vi "VAttrbutesToData.vi"(6 "to lowercase?(F)":bool, 7 "Prototype":variant, 8 "error in (no error)":errorcluster, 11 "VAttributes":variant) -> (0 "error out":errorcluster, 3 "data":variant)   [LabVIEW 2019, in "lv-apt-json-file.lvlib"]
uses:
  lv-apt-json-file.lvlib
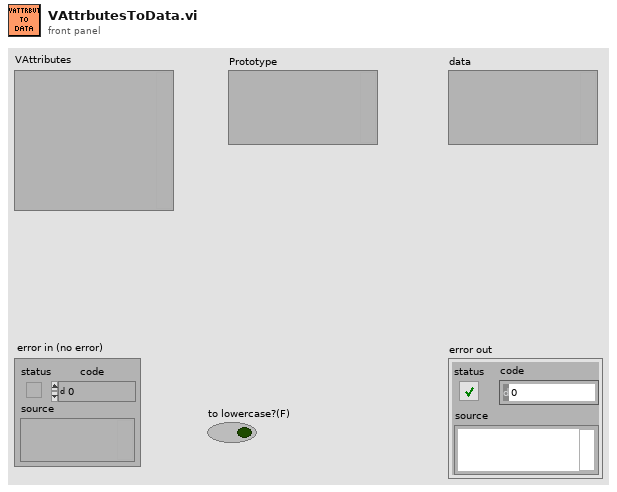
[diagram p1: front panel]
types:
  T1 = typedef "Type Descriptor Enumeration__ogtk.ctl" = enum8{"<Null>", "I8", "I16", "I32", "I64", "U8", "U16", "U32", "U64", "SGL", "DBL", "EXT", "CSG", "CDB", "CXT", "0x0F", "0x10", "0x11", "0x12", "0x13", "0x14", "Enum U8", "Enum U16", "Enum U32", "Enum U64", "SGL PQ", "DBL PQ", "EXT PQ", "CSG PQ", "CDB PQ", "CXT PQ", "0x1F", "0x20", "Boolean", "0x22", "0x23", "0x24", "0x25", "0x26", "0x27", "0x28", "0x29", "0x2A", "0x2B", "0x2C", "0x2D", "0x2E", "0x2F", "String", "0x31", "Path", "Pict", "0x34", "0x35", "0x36", "DAQ", "0x38", "0x39", "0x3A", "0x3B", "0x3C", "0x3D", "0x3E", "0x3F", "Array", "0x41", "0x42", "0x43", "0x44", "0x45", "0x46", "0x47", "0x48", "0x49", "0x4A", "0x4B", "0x4C", "0x4D", "0x4E", "0x4F", "Cluster", "0x51", "0x52", "Variant", "Waveform", "0x55", "0x56", "0x57", "0x58", "0x59", "0x5A", "0x5B", "0x5C", "0x5D", "0x5E", "Fixed Point", "0x60", "0x61", "0x62", "0x63", "0x64", "0x65", "0x66", "0x67", "0x68", "0x69", "0x6A", "0x6B", "0x6C", "0x6D", "0x6E", "0x6F", "Refnum", "0x71", "0x72", "Set Collection", "Map Collection"}
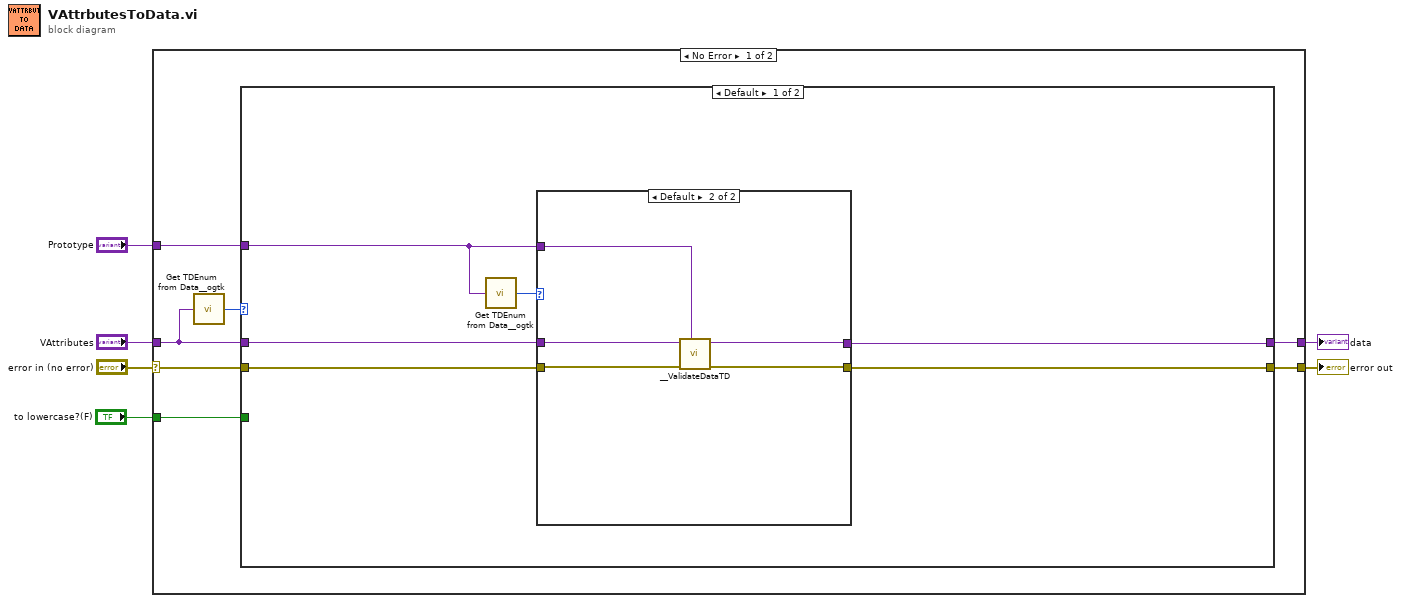
[diagram p0: block diagram]
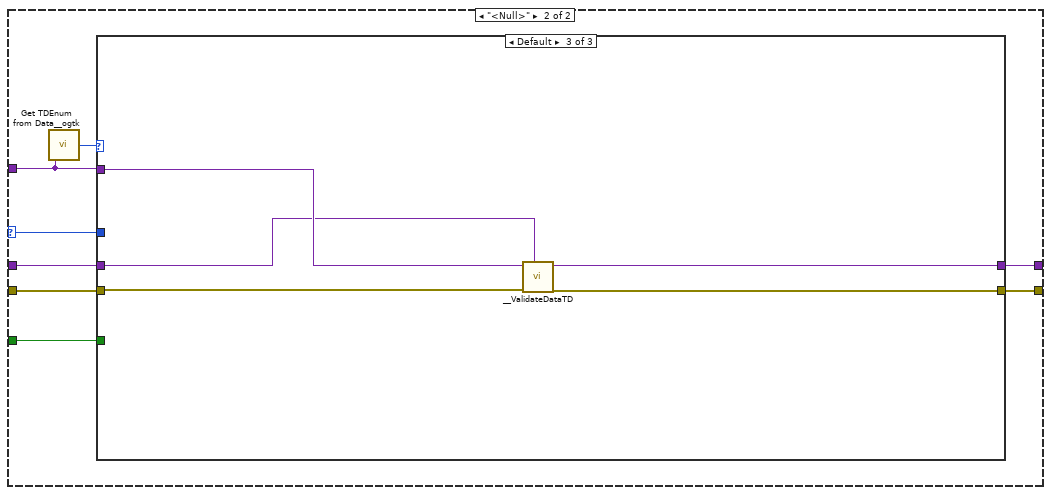
[diagram p3: hidden frame]
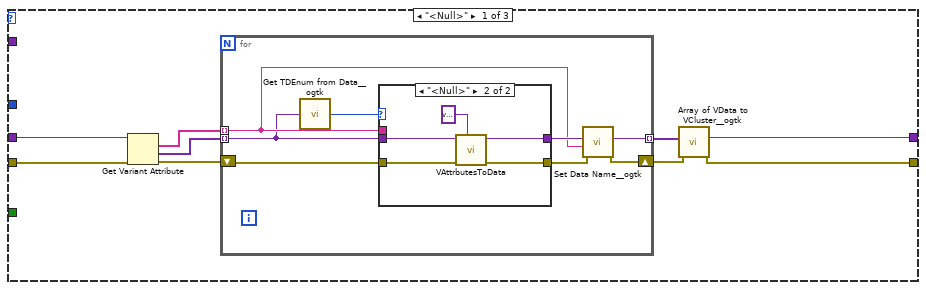
[diagram p4: hidden frame]
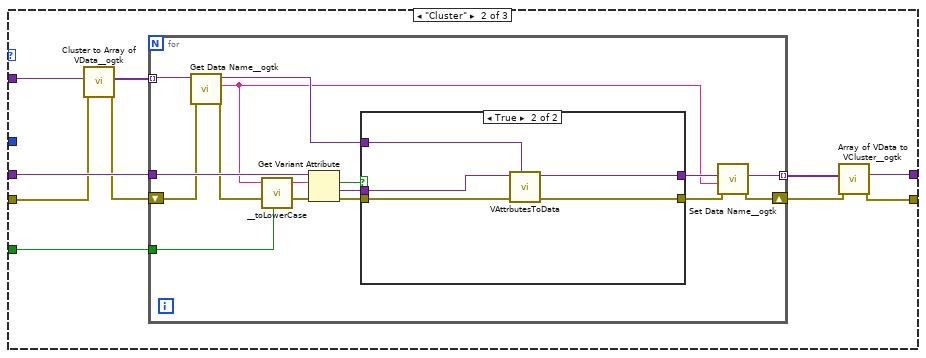
[diagram p6: hidden frame]
diagram:
  n1 = case shown="No Error" "error in (no error)" {
    selector: "error in (no error)" -> [w11 w96]
    tunnel: [w13 _] -> w6
    tunnel: [w12 w96] -> w5
    tunnel: "VAttributes" -> [w10 _]
    tunnel: "Prototype" -> [w8 _]
    tunnel: "to lowercase?(F)" -> [w7 _]
    frame No Error {
      n2 = call <userlib>:"Get TDEnum from Data__ogtk.vi"("Data"=w10) -> ("Type Descriptor Enumeration"=w9:T1)  [unwired: 4 in]
      n3 = case shown="Default" w9 {
        selector: w9 -> [_ w28]
        tunnel: [w18 w34] -> w13
        tunnel: [w19 w33] -> w12
        tunnel: w11 -> [w16 w32]
        tunnel: w8 -> [w14 w30]
        tunnel: w10 -> [w17 w29]
        tunnel: w7 -> [_ w27]
        frame Default {
          n4 = call <userlib>:"Get TDEnum from Data__ogtk.vi"("Data"=w14) -> ("Type Descriptor Enumeration"=w15:T1)  [unwired: 4 in]
          n5 = case shown="Default" w15 {
            tunnel: w16 -> [w20 w25]
            tunnel: [w20 w24] -> w19
            tunnel: w17 -> [w21 w26]
            tunnel: [w21 w23] -> w18
            tunnel: w14 -> [_ w22]
            frame "<Null>" {
            }
            frame Default {
              n6 = call "__ValidateDataTD.vi"("Expected Data"=w22, "error in (no error)"=w25, "Data"=w26) -> ("error out"=w24:errorcluster, "Data out"=w23:variant)  [unwired: 7 in]
            }
          }
        }
        frame "<Null>" {
          n7 = call <userlib>:"Get TDEnum from Data__ogtk.vi"("Data"=w30) -> ("Type Descriptor Enumeration"=w31:T1)  [unwired: 4 in]
          n8 = case shown="Default" w31 {
            tunnel: w29 -> [w40 w68 w91]
            tunnel: [w43 w67 w94] -> w34
            tunnel: [w42 w66 w92] -> w33
            tunnel: w32 -> [w41 w62 w93]
            tunnel: w30 -> [_ w63 w95]
            tunnel: w28 -> [_ _ _]
            tunnel: w27 -> [_ w59 _]
            frame "<Null>" {
              n9 = Get Variant Attribute(Variant=w40, error in=w41) -> (names=w38:string[], values=w39:variant[], error out=w36:errorcluster)  [unwired: 2 in, 1 out]
              n10 = for {
                tunnel: w39 -> [w45] mode=indexing
                tunnel: w38 -> [w48] mode=indexing
                tunnel: [w51] -> w37 mode=indexing
                shift-right: [w50] -> w35
                shift-left: w36 -> [w47]
                n11 = call <userlib>:"Get TDEnum from Data__ogtk.vi"("Data"=w45) -> ("Type Descriptor Enumeration"=w44:T1)  [unwired: 4 in]
                n12 = case shown="\"<Null>\"" w44 {
                  tunnel: w45 -> [w53 w58]
                  tunnel: [w53 w57] -> w49
                  tunnel: w48 -> [_ _]
                  tunnel: w47 -> [w52 w56]
                  tunnel: [w52 w55] -> w46
                  frame Default {
                  }
                  frame "<Null>" {
                    n13 = call "VAttrbutesToData.vi"("Prototype"=variant, "error in (no error)"=w56, "VAttributes"=w58) -> ("error out"=w55:errorcluster, "data"=w57:variant)  [unwired: 7 in]
                  }
                }
                n14 = call <userlib>:"Set Data Name__ogtk.vi"("error in (no error)"=w46, "Data Name"=w48, "Data"=w49) -> ("error out"=w50:errorcluster, "Renamed Data"=w51:variant)  [unwired: 7 in]
              }
              n15 = call <userlib>:"Array of VData to VCluster__ogtk.vi"("error in (no error)"=w35, "Array"=w37) -> ("error out"=w42:errorcluster, "VCluster"=w43:variant)  [unwired: 8 in]
            }
            frame "Cluster" {
              n16 = call <userlib>:"Cluster to Array of VData__ogtk.vi"("error in (no error)"=w62, "Cluster"=w63) -> ("error out"=w61:errorcluster, "Array of VData"=w60:variant[])  [unwired: 8 in]
              n17 = for {
                tunnel: w68 -> [w83]
                tunnel: [w82] -> w65 mode=indexing
                shift-right: [w80] -> w64
                shift-left: w61 -> [w73]
                tunnel: w60 -> [w77] mode=indexing
                tunnel: w59 -> [w69]
                n18 = call <userlib>:"Get Data Name__ogtk.vi"("error in (no error)"=w73, "Data"=w77) -> ("error out"=w72:errorcluster, "Data Name"=w71:string, "Data dup"=w75:variant)  [unwired: 7 in]
                n19 = call "__toLowerCase.vi"("Data Name in"=w71, "to lowercase?(F)"=w69) -> ("Data Name out"=w70:string)  [unwired: 5 in]
                n20 = Get Variant Attribute(Variant=w83, name=w70, error in=w72) -> (found=w76:bool, value=w74:variant, error out=w81:errorcluster)  [unwired: 1 in, 1 out]
                n21 = case shown="True" w76 {
                  tunnel: w81 -> [w84 w87]
                  tunnel: [w85 w88] -> w79
                  tunnel: [w84 w86] -> w78
                  tunnel: w75 -> [w85 w89]
                  tunnel: w74 -> [_ w90]
                  frame False {
                  }
                  frame True {
                    n22 = call "VAttrbutesToData.vi"("Prototype"=w89, "error in (no error)"=w87, "VAttributes"=w90) -> ("error out"=w86:errorcluster, "data"=w88:variant)  [unwired: 7 in]
                  }
                }
                n23 = call <userlib>:"Set Data Name__ogtk.vi"("error in (no error)"=w78, "Data Name"=w71, "Data"=w79) -> ("error out"=w80:errorcluster, "Renamed Data"=w82:variant)  [unwired: 7 in]
              }
              n24 = call <userlib>:"Array of VData to VCluster__ogtk.vi"("error in (no error)"=w64, "Array"=w65) -> ("error out"=w66:errorcluster, "VCluster"=w67:variant)  [unwired: 8 in]
            }
            frame Default {
              n25 = call "__ValidateDataTD.vi"("Expected Data"=w91, "error in (no error)"=w93, "Data"=w95) -> ("error out"=w92:errorcluster, "Data out"=w94:variant)  [unwired: 7 in]
            }
          }
        }
      }
    }
    frame Error {
    }
  }
  "data" <- w6
  "error out" <- w5
